vi "TIO Stream Read Non-blocking.vi"(8 "error in (no error)":errorcluster, 11 "TC Connection":T1={"Type"=enum."Serial", "URL"="serial:///dev/cu.usbserial-00000", "TO"=500, "Addr"=0, "Port"=0, "TCP"=refnum, "UDP"=refnum, "Route"=""}) -> (0 "error out":errorcluster, 1 "Payload":string, 2 "Type":u16(ring)=2 items=["Invalid", "Log", "RPC Request", "RPC Reply", "RPC Error", "Stream Description", "User"], 3 "TC Connection":T1={"Type"=enum."Serial", "URL"="serial:///dev/cu.usbserial-00000", "TO"=500, "Addr"=0, "Port"=0, "TCP"=refnum, "UDP"=refnum, "Route"=""}, 4 "Route":string, 5 "Routing Matches":bool)   [LabVIEW 2010]
uses:
  <userlib>/TIO Library 2010/TIO Serial Checksum CRC32.vi
panel:
  out "Routing Size":u8
  out "Payload Length":u16
  # "TODO Handle routing"
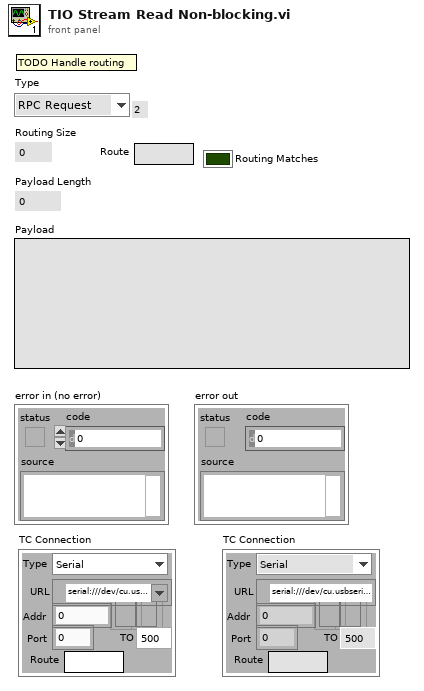
[diagram p1: front panel]
types:
  T1 = cluster{"Type":enum16{"Serial", "TCP", "UDP", "mUDP"}, "URL":refnum<visa-resource-name>, "TO":u32, "Addr":u32, "Port":i32, "TCP":refnum<k5>, "UDP":refnum<k16>, "Route":string}
  T2 = enum16{"Standard", "Buffered", "CRLF", "Immediate"}
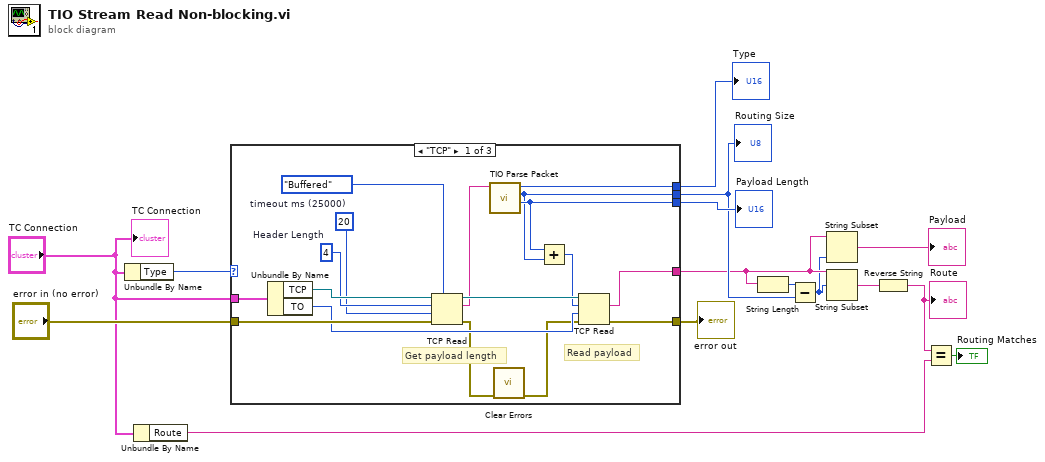
[diagram p0: block diagram]
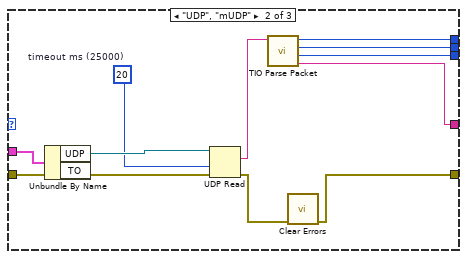
[diagram p2: hidden frame]
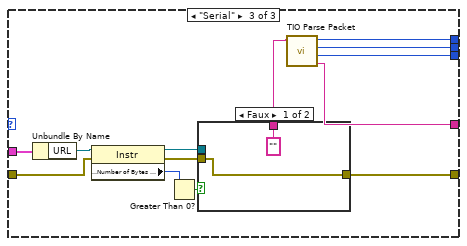
[diagram p3: hidden frame]
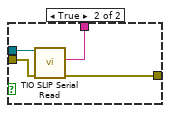
[diagram p4: hidden frame]
diagram:
  n1 = Unbundle By Name("TC Connection") -> ("Type"=w13:enum16{"Serial", "TCP", "UDP", "mUDP"})
  n2 = Unbundle By Name("TC Connection") -> ("Route"=w4:string)
  n3 = case shown="\"TCP\"" w13 {
    tunnel: "error in (no error)" -> [w29 w38 w47]
    tunnel: [w28 w33 w56] -> w15
    tunnel: "TC Connection" -> [w32 w43 w55]
    tunnel: [w27 w35 w51] -> w8
    tunnel: [w18 w41 w52] -> w12
    tunnel: [w17 w40 w53] -> w9
    tunnel: [w23 w42 w54] -> w11
    frame "TCP" {
      w22 = 20  # timeout ms (25000)
      w25 = u32 4  # Header Length
      # "Read payload"
      # "Get payload length"
      n4 = Unbundle By Name(w32) -> ("TCP"=w31:refnum<k5>, "TO"=w26:u32)
      n5 = TCP Read(connection ID=w31, bytes to read=w25, error in (no error)=w29, 7:T2."Buffered" ("mode (standard)"), 9:w22) -> (connection ID out=w30:refnum<k5>, data out=w24:string, error out=w20:errorcluster)
      n6 = call <userlib>:"TIO Parse Packet.vi"("Packet"=w24) -> ("Payload Length"=w18:u16, "Routing Size"=w17:u8, "Type"=w23:u16)  [unwired: 7 in, 1 out]
      n7 = call <vilib>:"Clear Errors.vi"("error in (no error)"=w20) -> ("error out"=w19:errorcluster)  [unwired: 6 in]
      n8 = Add(x=w18, y=w17) -> (x+y=w16:u16)
      n9 = TCP Read(connection ID=w30, bytes to read=w16, error in (no error)=w19, 9:w26) -> (data out=w27:string, error out=w28:errorcluster)  [unwired: 1 in, 1 out]
    }
    frame "UDP", "mUDP" {
      w37 = 20  # timeout ms (25000)
      n10 = Unbundle By Name(w43) -> ("UDP"=w39:refnum<k16>)  [unwired: 1 out]
      n11 = UDP Read(connection ID=w39, timeout ms (25000)=w37, 8:w38) -> (data out=w36:string, error out=w34:errorcluster)  [unwired: 1 in, 3 out]
      n12 = call <userlib>:"TIO Parse Packet.vi"("Packet"=w36) -> ("Payload"=w35:string, "Payload Length"=w41:u16, "Routing Size"=w40:u8, "Type"=w42:u16)  [unwired: 7 in]
      n13 = call <vilib>:"Clear Errors.vi"("error in (no error)"=w34) -> ("error out"=w33:errorcluster)  [unwired: 6 in]
    }
    frame "Serial" {
      n14 = Unbundle By Name(w55) -> ("URL"=w49:refnum<visa-resource-name>)
      n15 = property class="Instr"(reference=w49, error in=w47) -> (reference out=w48:refnum<visa-resource-name>, error out=w46:errorcluster, "Serial Settings:Number of Bytes at Serial Port"=w45:u32)
      n16 = Greater Than 0?(x=w45) -> (x > 0?=w44:bool)
      n17 = case shown="Faux" w44 {
        tunnel: [w58 w62] -> w56
        tunnel: ["" ("Payload") w61] -> w50
        tunnel: w48 -> [_ w60]
        tunnel: w46 -> [w58 w59]
        frame False {
        }
        frame True {
          n18 = call <userlib>:"TIO SLIP Serial Read.vi"("error in (no error)"=w59, "VISA resource name"=w60) -> ("error out"=w62:errorcluster, "Payload"=w61:string)  [unwired: 6 in, 2 out]
        }
      }
      n19 = call <userlib>:"TIO Parse Packet.vi"("Packet"=w50) -> ("Payload"=w51:string, "Payload Length"=w52:u16, "Routing Size"=w53:u8, "Type"=w54:u16)  [unwired: 7 in]
    }
  }
  "error out" <- w15
  "Type" <- w11
  "Routing Size" <- w9
  "Payload Length" <- w12
  n20 = String Length(string=w8) -> (length=w10:i32)
  n21 = Subtract(x=w10, y=w9) -> (x-y=w7:i32)
  n22 = String Subset(string=w8, length (rest)=w7) -> (substring=→"Payload":string)  [unwired: 1 in]
  n23 = String Subset(string=w8, offset (0)=w7) -> (substring=w2:string)  [unwired: 1 in]
  n24 = Reverse String(1:w2) -> (0:w1:string)
  "Route" <- w1
  n25 = Equal?(x=w1, y=w4) -> (x = y?=→"Routing Matches":bool)
  "TC Connection" <- "TC Connection"
